vi "Set Message2 Text.vi"(0 "handles cluster in":T2 caption="ハンドルクラスター入力", 5 "subject":string caption="件名", 7 "plain text message":string caption="標準テキストメッセージ", 11 "error in (no error)":errorcluster caption="エラー入力（エラーなし）", 12 "body charset (utf-8)":string="utf-8" caption="本文キャラセット (utf-8)", 13 "body transfer encoding (Base64)":T1(ring)=enum."Base64" caption="本文転送エンコーディング (Base64)") -> (4 "handles cluster out":T2 caption="ハンドルクラスター出力", 15 "error out":errorcluster caption="エラー出力")   [LabVIEW 2015]
doc: "Eメールの本文に含めるテキストを設定します。"
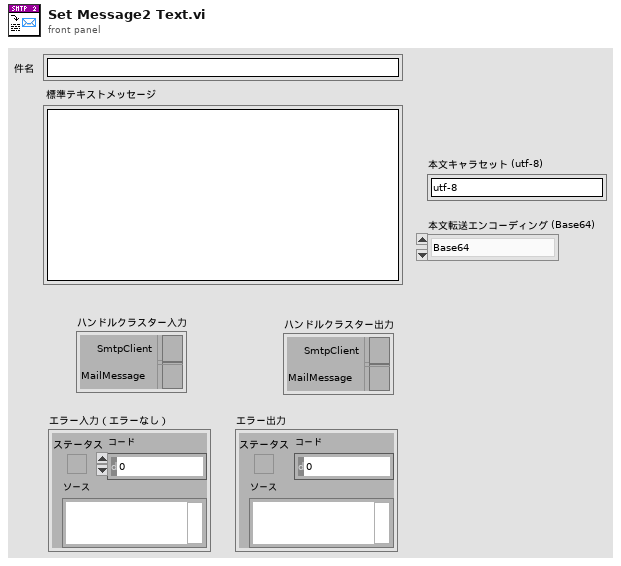
[diagram p1: front panel]
types:
  T1 = enum16{"QuotedPrintable", "Base64", "7bit", "8bit"}
  T2 = cluster{"SmtpClient":refnum<k24>, "MailMessage":refnum<k24>}
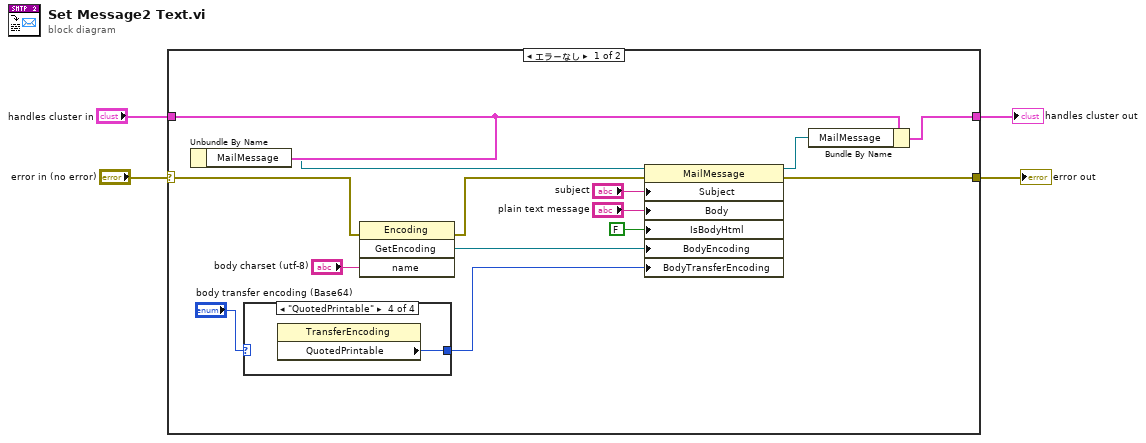
[diagram p0: block diagram]
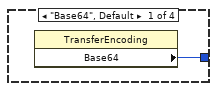
[diagram p2: hidden frame]
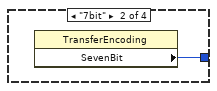
[diagram p3: hidden frame]
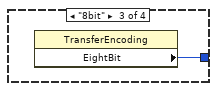
[diagram p4: hidden frame]
diagram:
  n1 = case shown="エラーなし" "error in (no error)" {
    selector: "error in (no error)" -> [w8 w24]
    tunnel: [w13 w24] -> w3
    tunnel: "handles cluster in" -> [w18 w23]
    tunnel: [w17 w23] -> w1
    frame No Error {
      n2 = Unbundle By Name(w18) -> ("MailMessage"=w16:refnum<k24>)
      n3 = case shown="\"QuotedPrintable\"" "body transfer encoding (Base64)" {
        tunnel: [w19 w20 w21 w22] -> w5
        frame "Base64", Default {
          n4 = property class="TransferEncoding"() -> ("Base64"=w19:i32)  [unwired: 2 in, 2 out]
        }
        frame "7bit" {
          n5 = property class="TransferEncoding"() -> ("SevenBit"=w20:i32)  [unwired: 2 in, 2 out]
        }
        frame "8bit" {
          n6 = property class="TransferEncoding"() -> ("EightBit"=w21:i32)  [unwired: 2 in, 2 out]
        }
        frame "QuotedPrintable" {
          n7 = property class="TransferEncoding"() -> ("QuotedPrintable"=w22:i32)  [unwired: 2 in, 2 out]
        }
      }
      n8 = invoke class="Encoding" method="GetEncoding"(error in=w8, "name"="body charset (utf-8)") -> (error out=w7:errorcluster, "GetEncoding"=w9:refnum<k24>)  [unwired: 2 in, 2 out]
      n9 = property class="MailMessage"(reference=w16, error in=w7, "Subject"="subject", "Body"="plain text message", "IsBodyHtml"=FALSE, "BodyEncoding"=w9, "BodyTransferEncoding"=w5) -> (reference out=w12:refnum<k24>, error out=w13:errorcluster)
      n10 = Bundle By Name(cluster=w18, "MailMessage"=w12) -> (w17:T2)
    }
    frame Error {
    }
  }
  "handles cluster out" <- w1
  "error out" <- w3
